vi "construct.vi"(8 "error in (no error)":errorcluster, 9 "configuration name":string, 10 "load config file?":bool=TRUE, 11 "DL090603DAQmxOnOffDetector in":refnum<class "DetectorDL090603DAQmxOnOff.lvclass">) -> (0 "error out":errorcluster, 3 "DL090603DAQmxOnOffDetector out":refnum<class "DetectorDL090603DAQmxOnOff.lvclass">)   [LabVIEW 2010, in "DetectorDL090603DAQmxOnOff.lvclass"]
uses:
  DetectorDL090603DAQmxOnOff.lvclass
  GenericDetector/GenericDetector/GenericDetector.lvclass
  DetectorDL090603DAQmxOnOff.lvclass/DetectorDL090603DAQmxOnOff.ctl
  DigitalOut/DigitalOutDL110325DAQmx/DigitalOutDL110325DAQmx/DigitalOutDL110325DAQmx.lvclass
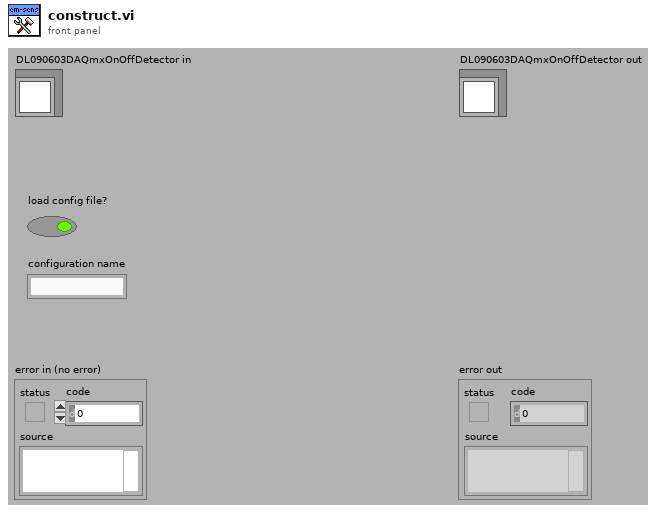
[diagram p1: front panel]
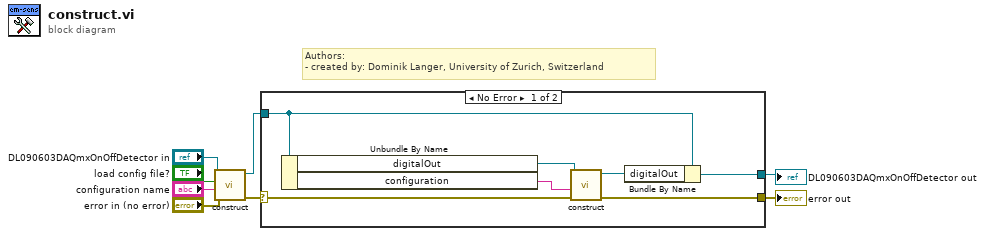
[diagram p0: block diagram]
diagram:
  # "Authors: \n- created by: Dominik Langer, University of Zurich, Switzerland"
  n1 = call-parent "construct.vi"("error in (no error)"="error in (no error)", "configuration name"="configuration name", "load config file?"="load config file?", "GenericPlugin in"="DL090603DAQmxOnOffDetector in") -> ("error out"=w4:errorcluster, "GenericPlugin out"=w3:refnum<class "DetectorDL090603DAQmxOnOff.lvclass">)  [unwired: 6 out]
  n2 = case shown="No Error" w4 {
    selector: w4 -> [w13 w16]
    tunnel: w3 -> [w15 w17]
    tunnel: [w14 w17] -> w2
    tunnel: [w12 w16] -> w1
    frame No Error {
      n3 = Unbundle By Name(w15) -> ("digitalOut"=w10:refnum<class "DigitalOutDL110325DAQmx.lvclass">, "configuration"=w11:string)
      n4 = call-dynamic "construct.vi"("error in (no error)"=w13, "configuration name"=w11, "GenericPlugin in"=w10) -> ("error out"=w12:errorcluster, "GenericPlugin out"=w9:refnum<class "DigitalOutDL110325DAQmx.lvclass">)  [unwired: 1 in, 6 out]
      n5 = Bundle By Name(cluster=w15, "digitalOut"=w9) -> (w14:refnum<class "DetectorDL090603DAQmxOnOff.lvclass">)
    }
    frame Error {
    }
  }
  "error out" <- w1
  "DL090603DAQmxOnOffDetector out" <- w2
